vi "Set Parameter.vi"(8 "error in (no error)":errorcluster, 10 "Parameter":refnum<class "Analyze Parameter Base.lvclass">, 11 "HIJ Vision Application in":refnum<class "HIJ Vision Application.lvclass">) -> (0 "error out":errorcluster, 3 "HIJ Vision Application out":refnum<class "HIJ Vision Application.lvclass">)   [LabVIEW 2014, in "HIJ Vision Application.lvlib" / "HIJ Vision Application.lvclass"]
uses:
  HIJ Vision Application.lvclass
  Analyze/Analyze Parameter/Analyze Parameter Base/Analyze Parameter Base.lvclass
  HIJ Vision Application.lvclass/HIJ Vision Application.ctl
  Analyze/Analyze Actor/Analyze Actor Messages/Set Analyze Parameter Msg/Set Analyze Parameter Msg.lvclass/Set Analyze Parameter Msg.ctl
  <vilib>/ActorFramework/Message Enqueuer/Message Enqueuer.lvclass/Message Enqueuer.ctl
  <vilib>/ActorFramework/Message Enqueuer/Enqueue.vi
  <vilib>/ActorFramework/Message Priority Queue/Priority Enqueue.vi
  Analyze/Analyze Actor/Analyze Actor Messages/Set Analyze Parameter Msg/Set Analyze Parameter Msg.lvclass
  Display Actors/HIJ Vision Display/HIJ Vision Display Messages/Evaluate with new Params Msg/Evaluate with new Params Msg.lvclass
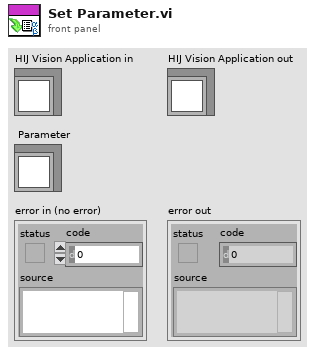
[diagram p1: front panel]
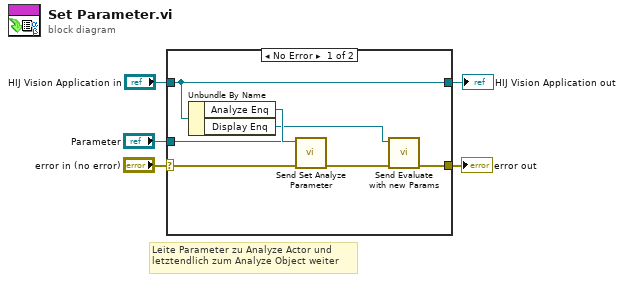
[diagram p0: block diagram]
diagram:
  # "Leite Parameter zu Analyze Actor und\nletztendlich zum Analyze Object weiter"
  n1 = case shown="No Error" "error in (no error)" {
    selector: "error in (no error)" -> [w9 w14]
    tunnel: [w6 w14] -> w4
    tunnel: [w12 w13] -> w2
    tunnel: "HIJ Vision Application in" -> [w12 w13]
    tunnel: "Parameter" -> [w10 _]
    frame No Error {
      n2 = Unbundle By Name(w12) -> ("Analyze Enq"=w11:refnum<class "Message Enqueuer.lvclass">, "Display Enq"=w8:refnum<class "Message Enqueuer.lvclass">)
      n3 = call "Send Set Analyze Parameter.vi"("error in (no error)"=w9, "Analyze Parameter"=w10, "Message Enqueuer"=w11) -> ("error out"=w7:errorcluster)  [unwired: 7 in, 1 out]
      n4 = call "Send Evaluate with new Params.vi"("error in (no error)"=w7, "Message Enqueuer"=w8) -> ("error out"=w6:errorcluster)  [unwired: 8 in, 1 out]
    }
    frame Error {
    }
  }
  "error out" <- w4
  "HIJ Vision Application out" <- w2
